vi "CH_LM Utility System Status.vi"(0 "Meter Index":i32, 5 "error in (no error)":errorcluster, 7 "Timeout / ms (3000)":i32=1000, 9 "Lock Timeout / ms (1000)":i32=1000) -> (11 "Lock timed out":bool, 14 "Meter Index":i32, 15 "System Status":T2 format="%.0x", 16 "Status":T1, 17 "Status Description":string, 19 "error out":errorcluster)   [LabVIEW 2012, in "CH_LM.lvlib"]
doc: "This query will get the system status. Status will be returned in a string expressed in upper case hexadecimal integer form. The 32-bit status word will be a bit-mapped status indicator. If a bit is set, the associated status will be active otherwise it will be inactive."
uses:
  CH_LM.lvlib
  CH_LM System Status.ctl
  CH_LM System StatusCluster.ctl
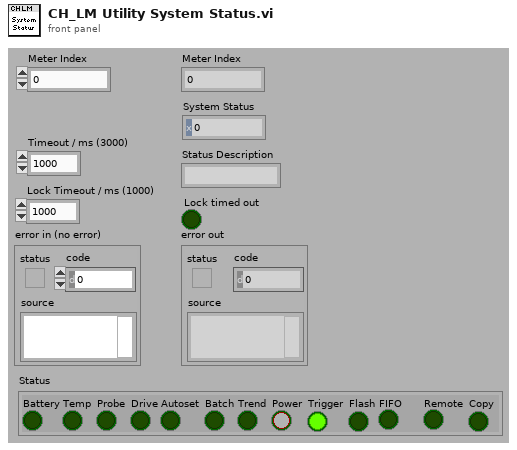
[diagram p1: front panel]
types:
  T1 = typedef "CH_LM.lvlib/CH_LM System StatusCluster.ctl" = cluster{"Battery":bool, "Temp":bool, "Probe":bool, "Drive":bool, "Autoset":bool, "Batch":bool, "Trend":bool, "Power":bool, "Trigger":bool, "Flash":bool, "FIFO":bool, "Remote":bool, "Copy":bool}
  T2 = typedef "CH_LM.lvlib/CH_LM System Status.ctl" = u32
  T3 = cluster{"[0]":bool, "[1]":bool, "[2]":bool, "[3]":bool, "[4]":bool, "[5]":bool, "[6]":bool, "[7]":bool, "[8]":bool, "[9]":bool, "[10]":bool, "[11]":bool, "[12]":bool}
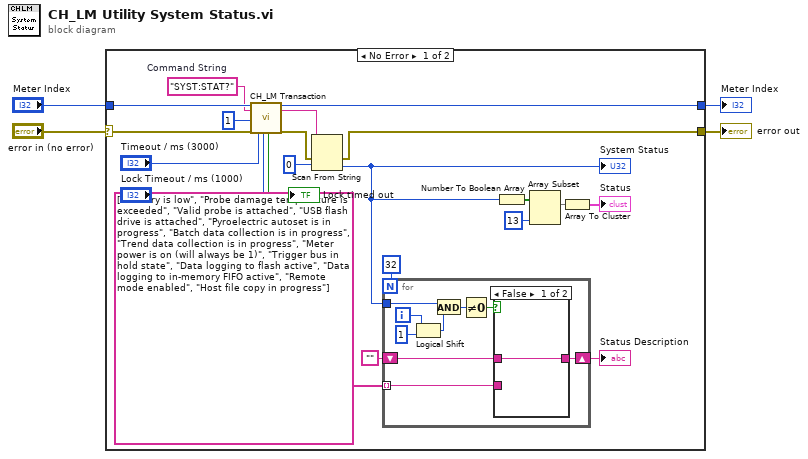
[diagram p0: block diagram]
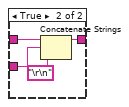
[diagram p2: hidden frame]
diagram:
  n1 = case shown="No Error" "error in (no error)" {
    selector: "error in (no error)" -> [w25 w41]
    tunnel: [w16 w41] -> w4
    tunnel: "Meter Index" -> [w24 w40]
    tunnel: [w23 w40] -> w1
    frame No Error {
      w18 = "SYST:STAT?"  # Command String
      n2 = call "CH_LM Transaction.vi"("Meter Index"=w24, "Command String"=w18, "NofStrings (-1:all)"=1 ("t"), "error in (no error)"=w25, "Timeout / ms (3000)"="Timeout / ms (3000)", "Lock Timeout / ms (1000)"="Lock Timeout / ms (1000)") -> ("Lock timed out"=→"Lock timed out":bool, "Meter Index"=w23:i32, "Response"=w15:string, "error out"=w17:errorcluster)  [unwired: 10 out]
      n3 = Scan From String(input string=w15, error in=w17, default 1=u32 0) -> (error out=w16:errorcluster, output 1=w6:u32)  [unwired: 2 in, 2 out]
      "System Status" <- w6
      n4 = for {
        N: 32 -> [_]
        tunnel: w6 -> [w32]
        shift-right: [w28] -> w10
        shift-left: "" -> [w30]
        tunnel: string[] ["Battery is low", "Probe damage temperature is exceeded", "Valid probe is attached", "USB flash drive is attached", "Pyroelectric autoset is in progress", "Batch data collection is in progress", "Trend data collection is in progress", "Meter power is on (will always be 1)", "Trigger bus in hold state", "Data logging to flash active", "Data logging to in-memory FIFO active", "Remote mode enabled", "Host file copy in progress"] -> [w29] mode=indexing
        i -> [w33]
        n5 = Logical Shift(y=w33, x=u32 1) -> (x << y=w31:u32)
        n6 = And(x=w32, y=w31) -> (x .and. y?=w27:u32)
        n7 = Not Equal To 0?(x=w27) -> (x != 0?=w26:bool)
        n8 = case shown="False" w26 {
          tunnel: w30 -> [w35 w39]
          tunnel: w29 -> [_ w37]
          tunnel: [w35 w38] -> w28
          frame False {
          }
          frame True {
            n9 = Concatenate Strings(w39, w37, "\r\n") -> (w38:string)
          }
        }
      }
      "Status Description" <- w10
      n10 = Number To Boolean Array(number=w6) -> (Boolean array=w5:bool[])
      n11 = Array Subset(array=w5, length=13) -> (w7:bool[])  [unwired: 1 in]
      n12 = Array To Cluster(array=w7) -> (cluster=→"Status":T3)
    }
    frame Error {
    }
  }
  "error out" <- w4
  "Meter Index" <- w1
